vi "VNA GetData.vi"(8 "error in (no error)":errorcluster, 9 "command delay (ms)":u32=1000, 10 "Trace Name":T1, 11 "LibreVNA in":refnum<class "LibreVNA.lvclass">) -> (0 "error out":errorcluster, 1 "Data Out":dbl[][](array[numeric]), 2 "Recv Buffer":string, 3 "LibreVNA out":refnum<class "LibreVNA.lvclass">, 4 "rows":i32, 5 "TimeStamp":timestamp)   [LabVIEW 2023, in "LibreVNA.lvclass"]
uses:
  LibreVNA.lvclass
  Types/Trace Enum.ctl
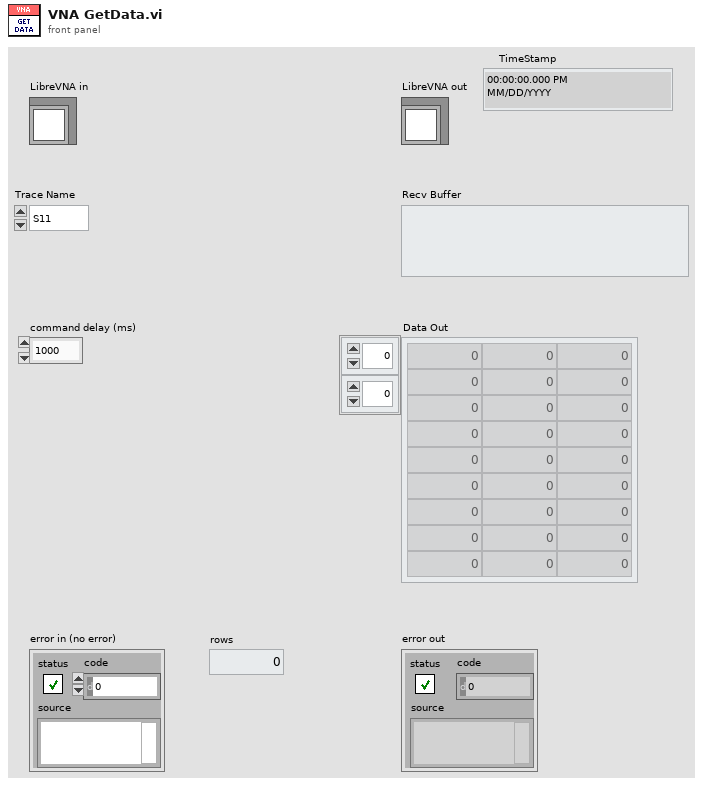
[diagram p1: front panel]
types:
  T1 = typedef "LibreVNA.lvclass/Trace Enum.ctl" = enum16{"S11", "S12", "S21", "S22"}
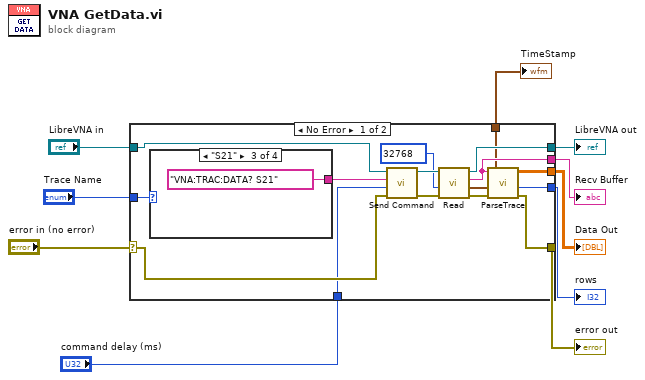
[diagram p0: block diagram]
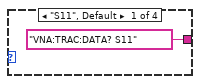
[diagram p2: hidden frame]
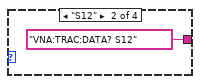
[diagram p3: hidden frame]
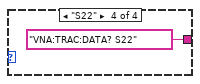
[diagram p4: hidden frame]
diagram:
  n1 = case shown="No Error" "error in (no error)" {
    selector: "error in (no error)" -> [w21 w31]
    tunnel: [w16 w31] -> w9
    tunnel: [w20 w30] -> w7
    tunnel: "LibreVNA in" -> [w25 w30]
    tunnel: "Trace Name" -> [w24 _]
    tunnel: [w15 _] -> w5
    tunnel: [w14 _] -> w4
    tunnel: [w13 _] -> w3
    tunnel: "command delay (ms)" -> [w12 _]
    tunnel: [w11 _] -> w1
    frame No Error {
      n2 = case shown="\"S21\"" w24 {
        tunnel: ["VNA:TRAC:DATA? S11" "VNA:TRAC:DATA? S12" "VNA:TRAC:DATA? S21" "VNA:TRAC:DATA? S22"] -> w22
        frame "S11", Default {
        }
        frame "S12" {
        }
        frame "S21" {
        }
        frame "S22" {
        }
      }
      n3 = call-dynamic "Send Command.vi"("error in (no error)"=w21, "command delay (ms)"=w12, "Command"=w22, "LibreVNA in"=w25) -> ("error out"=w19:errorcluster, "LibreVNA out"=w23:refnum<class "LibreVNA.lvclass">)  [unwired: 5 in, 1 out]
      n4 = call-dynamic "Read.vi"("error in (no error)"=w19, "bytes to read"=32768, "LibreVNA in"=w23) -> ("error out"=w17:errorcluster, "TimeStamp"=w11:timestamp, "Recv Buffer"=w14:string, "LibreVNA out"=w20:refnum<class "LibreVNA.lvclass">)  [unwired: 5 in]
      n5 = call "ParseTrace.vi"("error in"=w17, "Buffer in"=w14) -> ("error out"=w16:errorcluster, "rows"=w13:i32, "Data Out"=w15:dbl[][])  [unwired: 3 in]
    }
    frame Error {
    }
  }
  "error out" <- w9
  "LibreVNA out" <- w7
  "Data Out" <- w5
  "Recv Buffer" <- w4
  "rows" <- w3
  "TimeStamp" <- w1
